vi "RunInferenceAllOutput.vi"(8 "error in (no error)":errorcluster, 11 "ONNX Class in":refnum<class "ONNX Class.lvclass">) -> (0 "error out":errorcluster, 2 "Output Buffer":sgl[](array[numeric]), 3 "ONNX Class out":refnum<class "ONNX Class.lvclass">)   [LabVIEW 2017, in "ONNX Class Library.lvlib" / "ONNX Class.lvclass"]
uses:
  ONNX Class.lvclass
  ONNX Class.lvclass/ONNX Class.ctl
  ONNX Class Library.lvlib
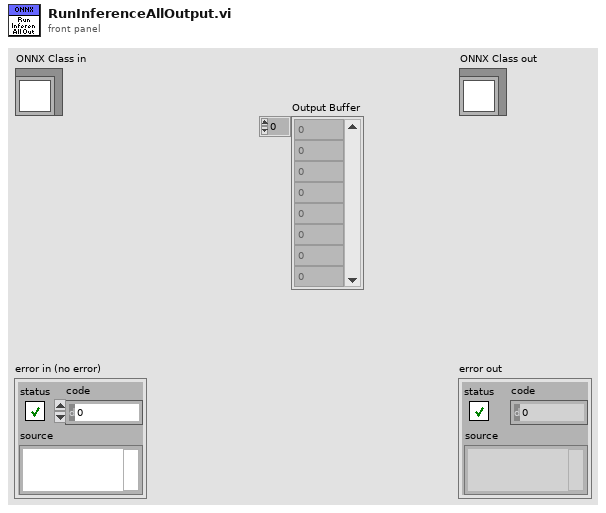
[diagram p1: front panel]
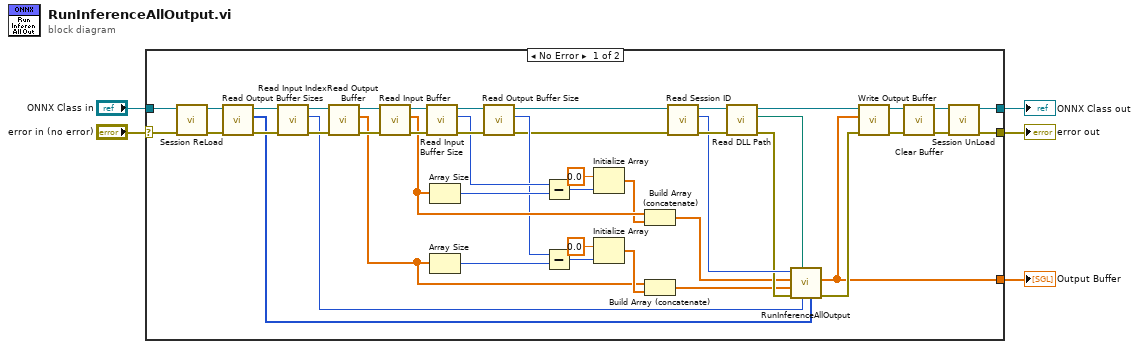
[diagram p0: block diagram]
diagram:
  n1 = case shown="No Error" "error in (no error)" {
    selector: "error in (no error)" -> [w49 w53]
    tunnel: [w41 w53] -> w4
    tunnel: [w42 w52] -> w2
    tunnel: "ONNX Class in" -> [w50 w52]
    tunnel: [w28 _] -> w1
    frame No Error {
      n2 = call-dynamic "Session ReLoad.vi"("error in (no error)"=w49, "ONNX Class in"=w50) -> ("error out"=w37:errorcluster, "ONNX Class out"=w38:refnum<class "ONNX Class.lvclass">)  [unwired: 8 in]
      n3 = call-dynamic "Read Output Buffer Sizes.vi"("error in (no error)"=w37, "ONNX Class in"=w38) -> ("error out"=w35:errorcluster, "Output Buffer Sizes"=w6:i32[], "ONNX Class out"=w36:refnum<class "ONNX Class.lvclass">)  [unwired: 7 in]
      n4 = call-dynamic "Read Input Index.vi"("error in (no error)"=w35, "ONNX Class in"=w36) -> ("error out"=w33:errorcluster, "Input Index"=w7:i32, "ONNX Class out"=w34:refnum<class "ONNX Class.lvclass">)  [unwired: 7 in]
      n5 = call-dynamic "Read Output Buffer.vi"("error in (no error)"=w33, "ONNX Class in"=w34) -> ("error out"=w39:errorcluster, "Output Buffer"=w16:sgl[], "ONNX Class out"=w40:refnum<class "ONNX Class.lvclass">)  [unwired: 7 in]
      n6 = call-dynamic "Read Input Buffer.vi"("error in (no error)"=w39, "ONNX Class in"=w40) -> ("error out"=w29:errorcluster, "Input Buffer"=w23:sgl[], "ONNX Class out"=w32:refnum<class "ONNX Class.lvclass">)  [unwired: 7 in]
      n7 = call-dynamic "Read Input Buffer Size.vi"("error in (no error)"=w29, "ONNX Class in"=w32) -> ("error out"=w30:errorcluster, "Input Buffer Size"=w26:i64, "ONNX Class out"=w31:refnum<class "ONNX Class.lvclass">)  [unwired: 7 in]
      n8 = Array Size(array=w23) -> (size(s)=w27:i32)
      n9 = Array Size(array=w16) -> (size(s)=w17:i32)
      n10 = call-dynamic "Read Output Buffer Size.vi"("error in (no error)"=w30, "ONNX Class in"=w31) -> ("error out"=w9:errorcluster, "Output Buffer Size"=w15:i64, "ONNX Class out"=w10:refnum<class "ONNX Class.lvclass">)  [unwired: 7 in]
      n11 = Subtract(x=w26, y=w27) -> (x-y=w25:i64)
      n12 = Subtract(x=w15, y=w17) -> (x-y=w18:i64)
      n13 = Initialize Array(sgl 0.0 ("element"), w25) -> (w22:sgl[])
      n14 = Initialize Array(sgl 0.0 ("element"), w18) -> (w20:sgl[])
      n15 = Build Array (concatenate)(w23, w22) -> (w21:sgl[])
      n16 = Build Array (concatenate)(w16, w20) -> (w8:sgl[])
      n17 = call-dynamic "Read Session ID.vi"("error in (no error)"=w9, "ONNX Class in"=w10) -> ("error out"=w47:errorcluster, "Session ID"=w46:i32, "ONNX Class out"=w48:refnum<class "ONNX Class.lvclass">)  [unwired: 7 in]
      n18 = call-dynamic "Read DLL Path.vi"("error in (no error)"=w47, "ONNX Class in"=w48) -> ("error out"=w45:errorcluster, "DLL Path"=w44:path, "ONNX Class out"=w43:refnum<class "ONNX Class.lvclass">)  [unwired: 7 in]
      n19 = call "RunInferenceAllOutput.vi"("outputSizes"=w6, "inputIndex"=w7, "DLL path"=w44, "error in (no error)"=w45, "outputBuffer in"=w8, "inputBuffer"=w21, "session id in"=w46) -> ("error out"=w51:errorcluster, "outputBuffer"=w28:sgl[])  [unwired: 2 in, 1 out]
      n20 = call-dynamic "Write Output Buffer.vi"("error in (no error)"=w51, "Output Buffer"=w28, "ONNX Class in"=w43) -> ("error out"=w13:errorcluster, "ONNX Class out"=w14:refnum<class "ONNX Class.lvclass">)  [unwired: 7 in]
      n21 = call-dynamic "Clear Buffer.vi"("error in (no error)"=w13, "ONNX Class in"=w14) -> ("error out"=w11:errorcluster, "ONNX Class out"=w12:refnum<class "ONNX Class.lvclass">)  [unwired: 8 in]
      n22 = call-dynamic "Session UnLoad.vi"("error in (no error)"=w11, "ONNX Class in"=w12) -> ("error out"=w41:errorcluster, "ONNX Class out"=w42:refnum<class "ONNX Class.lvclass">)  [unwired: 8 in]
    }
    frame Error {
    }
  }
  "error out" <- w4
  "ONNX Class out" <- w2
  "Output Buffer" <- w1
